vi "test Add-Find-Remove.vi"(8 "error in":errorcluster, 11 "TestCase in":refnum<class "Scripting.lvclass">) -> (0 "error out":errorcluster, 3 "TestCase out":refnum<class "Scripting.lvclass">)   [LabVIEW 2020, in "Scripting.lvclass"]
uses:
  Scripting.lvclass
  <vilib>/addons/_JKI Toolkits/VI Tester/TestCase.llb/TestCase.lvclass
  Scripting/Ballard MIL-STD-1553 Scripting.lvlib
  C:/Git/niveristand-custom-device-testing-tools/VeriStandScriptingTestCase/VeriStandScriptingTestCase.lvclass
  C:/Program Files (x86)/National Instruments/LabVIEW 2020/vi.lib/addons/_JKI Toolkits/VI Tester/TestCase.llb/TestCase.lvclass
  C:/Git/niveristand-ballard-milStd1553-custom-device/Source/Custom Device Support/Tests/Unit/Scripting/Scripting.lvclass
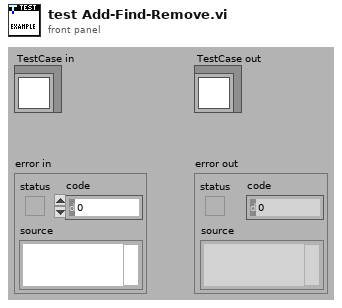
[diagram p1: front panel]
types:
  T1 = typedef "Custom Device API.lvlib/Custom Device Item Ref.ctl" = u64
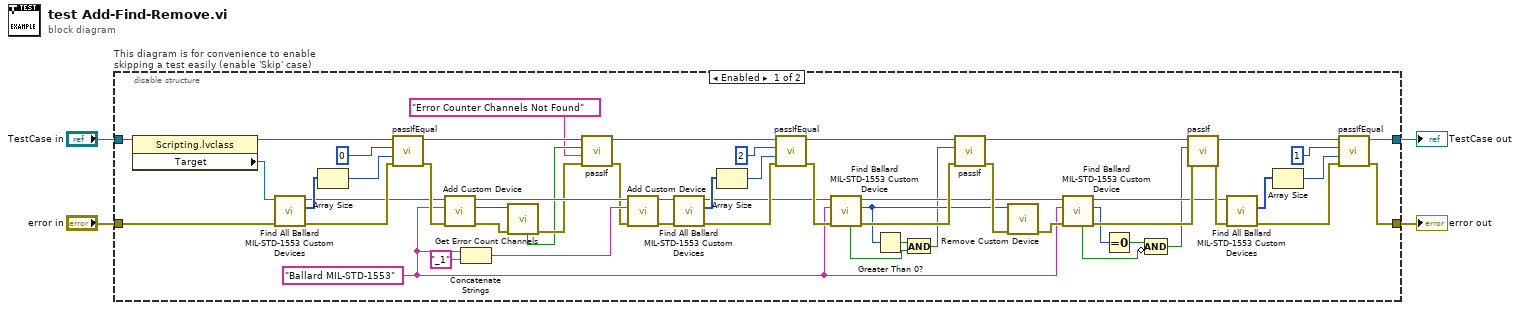
[diagram p0: block diagram]
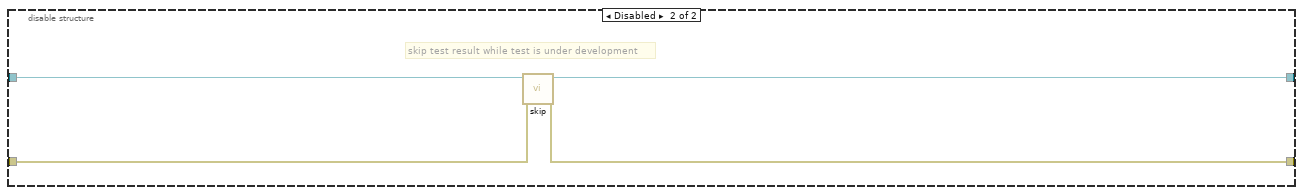
[diagram p2: hidden frame]
diagram:
  n1 = disable-structure "This diagram is for convenience to enable skipping a test easily (enable 'Skip' case)" shown="Enabled" {
    disable-tunnel: "TestCase in" -> [w23 w62]
    disable-tunnel: [w26 w60] -> w1
    disable-tunnel: [w25 w61] -> w3
    disable-tunnel: "error in" -> [w58 w59]
    frame Enabled {
      w36 = "Ballard MIL-STD-1553" ("name")
      n2 = property class="Scripting.lvclass"(reference=w23) -> (reference out=w21:refnum<class "Scripting.lvclass">, "Target"=w22:refnum<k24>)  [unwired: 1 in, 1 out]
      n3 = call "Find All Ballard MIL-STD-1553 Custom Devices.vi"("error in"=w58, "target in"=w22) -> ("error out"=w54:errorcluster, "Ballard MIL-STD-1553 custom devices"=w57:T1[], "target out"=w52:refnum<k24>)  [unwired: 7 in]
      n4 = Array Size(array=w57) -> (size(s)=w56:i32)
      n5 = call-dynamic "passIfEqual.vi"("error in (no error)"=w54, "y"=w56, "x"=0 ("size(s)"), "TestCase in"=w21) -> ("error out"=w53:errorcluster, "TestCase out"=w18:refnum<class "Scripting.lvclass">)  [unwired: 6 in]
      n6 = call "Add Custom Device.vi"("error in"=w53, "name"=w36, "target in"=w52) -> ("error out"=w19:errorcluster, "Ballard MIL-STD 1553 custom device"=w20:T1, "target out"=w50:refnum<k24>)  [unwired: 6 in]
      n7 = Concatenate Strings(w36, "_1" ("string")) -> (w49:string)
      n8 = call "Get Error Count Channels.vi"("error in"=w19, "Ballard MIL-STD-1553 custom device in"=w20) -> ("error out"=w16:errorcluster, "found?"=w14:bool)  [unwired: 6 in, 2 out]
      n9 = call-dynamic "passIf.vi"("error in (no error)"=w16, "message (\"\")"="Error Counter Channels Not Found" ("message (\"\")"), "pass"=w14, "TestCase in"=w18) -> ("error out"=w15:errorcluster, "TestCase out"=w17:refnum<class "Scripting.lvclass">)  [unwired: 6 in]
      n10 = call "Add Custom Device.vi"("error in"=w15, "name"=w49, "target in"=w50) -> ("error out"=w48:errorcluster, "target out"=w47:refnum<k24>)  [unwired: 6 in, 1 out]
      n11 = call "Find All Ballard MIL-STD-1553 Custom Devices.vi"("error in"=w48, "target in"=w47) -> ("error out"=w43:errorcluster, "Ballard MIL-STD-1553 custom devices"=w44:T1[], "target out"=w41:refnum<k24>)  [unwired: 7 in]
      n12 = Array Size(array=w44) -> (size(s)=w45:i32)
      n13 = call-dynamic "passIfEqual.vi"("error in (no error)"=w43, "y"=w45, "x"=2 ("size(s)"), "TestCase in"=w17) -> ("error out"=w42:errorcluster, "TestCase out"=w40:refnum<class "Scripting.lvclass">)  [unwired: 6 in]
      n14 = call "Find Ballard MIL-STD-1553 Custom Device.vi"("error in"=w42, "name"=w36, "target in"=w41) -> ("error out"=w39:errorcluster, "Ballard MIL-STD 1553 custom device"=w11:T1, "target out"=w35:refnum<k24>, "found?"=w8:bool)  [unwired: 5 in]
      n15 = Greater Than 0?(x=w11) -> (x > 0?=w12:bool)
      n16 = And(x=w12, y=w8) -> (x .and. y?=w9:bool)
      n17 = call-dynamic "passIf.vi"("error in (no error)"=w39, "pass"=w9, "TestCase in"=w40) -> ("error out"=w38:errorcluster, "TestCase out"=w34:refnum<class "Scripting.lvclass">)  [unwired: 7 in]
      n18 = call "Remove Custom Device.vi"("error in"=w38, "Ballard MIL-STD 1553 custom device"=w11) -> ("error out"=w37:errorcluster)  [unwired: 9 in]
      n19 = call "Find Ballard MIL-STD-1553 Custom Device.vi"("error in"=w37, "name"=w36, "target in"=w35) -> ("error out"=w33:errorcluster, "Ballard MIL-STD 1553 custom device"=w10:T1, "target out"=w31:refnum<k24>, "found?"=w7:bool)  [unwired: 5 in]
      n20 = Equal To 0?(x=w10) -> (x = 0?=w6:bool)
      n21 = Compound Arithmetic op=AND(w6, invert w7) -> (w5:bool)
      n22 = call-dynamic "passIf.vi"("error in (no error)"=w33, "pass"=w5, "TestCase in"=w34) -> ("error out"=w32:errorcluster, "TestCase out"=w29:refnum<class "Scripting.lvclass">)  [unwired: 7 in]
      n23 = call "Find All Ballard MIL-STD-1553 Custom Devices.vi"("error in"=w32, "target in"=w31) -> ("error out"=w28:errorcluster, "Ballard MIL-STD-1553 custom devices"=w27:T1[])  [unwired: 7 in, 1 out]
      n24 = Array Size(array=w27) -> (size(s)=w24:i32)
      n25 = call-dynamic "passIfEqual.vi"("error in (no error)"=w28, "y"=w24, "x"=1 ("size(s)"), "TestCase in"=w29) -> ("error out"=w25:errorcluster, "TestCase out"=w26:refnum<class "Scripting.lvclass">)  [unwired: 6 in]
    }
    frame Disabled {
      # "skip test result while test is under development"
      n26 = call <vilib>:"skip.vi"("error in (no error)"=w59, "TestCase in"=w62) -> ("error out"=w61:errorcluster, "TestCase out"=w60:refnum<class "Scripting.lvclass">)  [unwired: 8 in]
    }
  }
  "error out" <- w3
  "TestCase out" <- w1
